vi "Single Side Real FFT PtByPt.vi"(4 "initialize":bool, 5 "sample length":i32=100, 8 "input data":dbl format="%0.2f") -> (0 "error":i32, 1 "half length":i32, 2 "sample length":i32, 3 "FFT Single Side":cdb[](array[numeric]) format="%0.2f")   [LabVIEW 2020, in "NI_PtbyPt.lvlib"]
uses:
  <vilib>/ptbypt/NI_PtbyPt.lvlib
  <vilib>/Analysis/1siggen.llb/Ramp Pattern by Samples.vi
  <vilib>/Analysis/NI_AALBase.lvlib
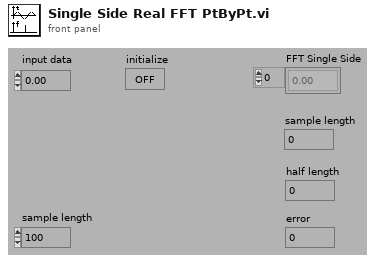
[diagram p1: front panel]
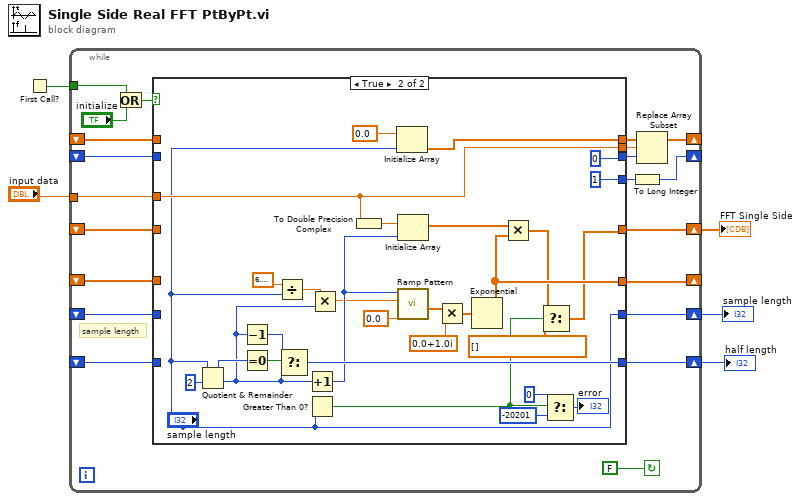
[diagram p0: block diagram]
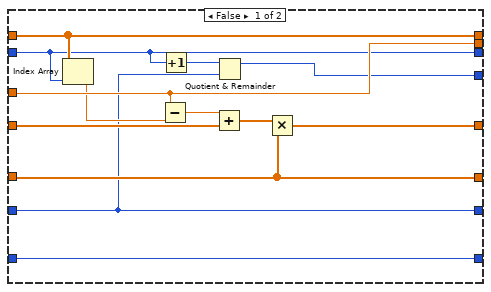
[diagram p2: hidden frame]
diagram:
  n1 = First Call?() -> (First Call?: T/F=w5:bool)
  n2 = while {
    tunnel: w5 -> [w8]
    shift-left: _ -> [w11]
    shift-right: [w10] -> w1
    shift-left: _ -> [w14]
    shift-right: [w15] -> w3
    shift-left: _ -> [w17]
    shift-right: [w16] -> _
    shift-left: _ -> [w22]
    shift-right: [w23] -> _
    tunnel: "input data" -> [w12]
    shift-left: _ -> [w24]
    shift-right: [w26] -> w4
    shift-left: _ -> [w25]
    shift-right: [w20] -> _
    stop <- FALSE continue-if-true
    # "sample length"
    n3 = Or(x=w8, y="initialize") -> (x .or. y?=w6:bool)
    n4 = case shown="True" w6 {
      tunnel: w12 -> [w38 w61]
      tunnel: w11 -> [w29 _]
      tunnel: [w31 w40] -> w26
      tunnel: [w39 w68] -> w21
      tunnel: w25 -> [w39 _]
      tunnel: w24 -> [w34 _]
      tunnel: [w32 w53] -> w23
      tunnel: w22 -> [w32 _]
      tunnel: [w30 0 ("Index")] -> w19
      tunnel: [w27 1 ("Index")] -> w18
      tunnel: w17 -> [w30 _]
      tunnel: w14 -> [w35 _]
      tunnel: [w35 w55] -> w15
      tunnel: [w38 w61] -> w13
      tunnel: [w29 "sample length"] -> w10
      frame False {
        n5 = Index Array(array=w39, index=w30) -> (element=w37:dbl)
        n6 = Subtract(x=w38, y=w37) -> (x-y=w36:dbl)
        n7 = Increment(x=w30) -> (x+1=w28:i32)
        n8 = Add(x=w36, y=w34) -> (x+y=w33:cdb[])
        n9 = Quotient & Remainder(x=w28, y=w29) -> (x-y*floor(x/y)=w27:i32)  [unwired: 1 out]
        n10 = Multiply(x=w33, y=w32) -> (x*y=w31:cdb[])
      }
      frame True {
        n11 = Quotient & Remainder(x="sample length", y=2) -> (x-y*floor(x/y)=w58:i32, floor(x/y)=w48:i32)
        n12 = Decrement(x=w48) -> (x-1=w56:i32)
        n13 = Equal To 0?(x=w58) -> (x = 0?=w57:bool)
        n14 = Divide(x=6.283185307179586, y="sample length") -> (x/y=w51:dbl)
        n15 = Select(t=w56, s=w57, f=w48) -> (s? t:f=w55:i32)
        n16 = Increment(x=w48) -> (x+1=w50:i32)
        n17 = Greater Than 0?(x="sample length") -> (x > 0?=w43:bool)
        n18 = Multiply(x=w51, y=w48) -> (x*y=w49:dbl)
        n19 = To Double Precision Complex(1:w61) -> (0:w60:cdb)
        n20 = Initialize Array(0.0 ("Element Data"), "sample length") -> (w68:dbl[])
        n21 = Initialize Array(w60, w50) -> (w54:cdb[])
        n22 = call-poly <vilib>:"Ramp Pattern.vi"("start"=0.0, "end"=w49, "samples"=w50) -> ("Ramp Pattern"=w63:dbl[])  [unwired: 7 in, 1 out]
        n23 = Multiply(x=w63, y=cdb 0.0+1.0i) -> (x*y=w67:cdb[])
        n24 = Exponential(1:w67) -> (0:w53:cdb[])
        n25 = Multiply(x=w54, y=w53) -> (x*y=w42:cdb[])
        n26 = Select(t=w42, s=w43, f=cdb[] []) -> (s? t:f=w40:cdb[])
        n27 = Select(t=0, s=w43, f=-20201) -> (s? t:f=→"error":i32)
      }
    }
    n28 = To Long Integer(number=w18) -> (32bit integer=w16:i32)
    n29 = Replace Array Subset(array=w21, new element=w13, index=w19) -> (w20:dbl[])
  }
  "FFT Single Side" <- w4
  "half length" <- w3
  "sample length" <- w1
